vi "2.1 Helper - LatLong to UTM.vi"(1 "East/West":string, 2 "Longitude":dbl, 3 "North/South":string, 4 "Latitude":dbl) -> (0 "Robot UTM Location":T1)   [LabVIEW 2011]
uses:
  2 Typedefs/UTM Location.ctl
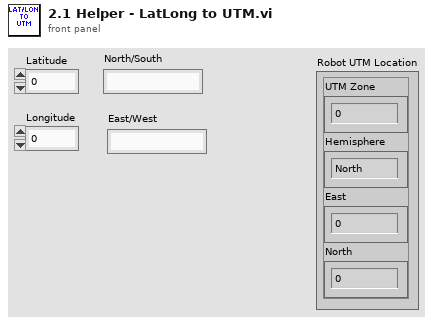
[diagram p1: front panel]
types:
  T1 = typedef "UTM Location.ctl" = cluster{"UTM Zone":dbl, "Hemisphere":enum16{"North", "South"}, "East":dbl, "North":dbl}
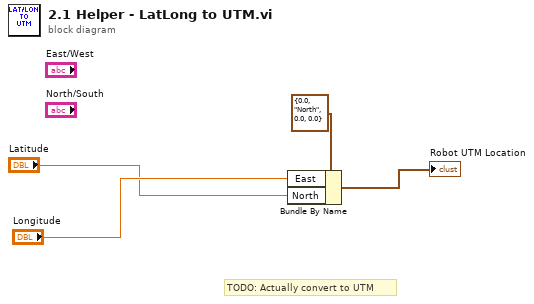
[diagram p0: block diagram]
diagram:
  # "TODO: Actually convert to UTM"
  n1 = Bundle By Name(cluster=T1 {"UTM Zone"=0.0, "Hemisphere"=enum."North", "East"=0.0, "North"=0.0} ("Robot UTM Location"), "East"="Longitude", "North"="Latitude") -> (→"Robot UTM Location":T1)
